vi "piezoDoubleDynReg.vi"   [LabVIEW 2017]
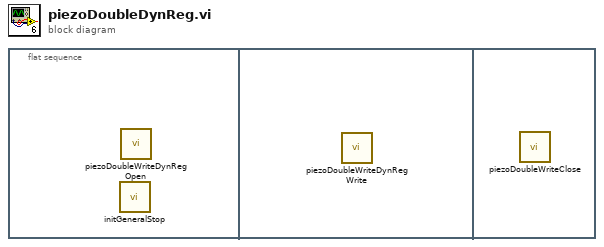
[diagram p0: block diagram]
diagram:
  n1 = flat-sequence {
    frame #0 {
      n2 = call "initGeneralStop.vi"() -> ()  [unwired: 1 in]
      n3 = call "piezoDoubleWriteDynRegOpen.vi"() -> ()  [unwired: 12 in]
    }
    frame #1 {
      n4 = call "piezoDoubleWriteDynRegWrite.vi"() -> ()  [unwired: 12 in]
    }
    frame #2 {
      n5 = call "piezoDoubleWriteClose.vi"() -> ()  [unwired: 1 in]
    }
  }
